vi "API Test.vi"   [LabVIEW 2020]
uses:
  <userlib>/_MGI/User Interface/Progress Bar/Progress Bar.lvclass
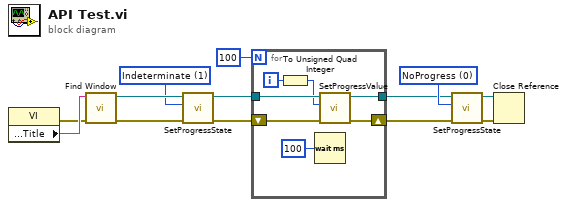
[diagram p0: block diagram]
diagram:
  w12 = 0 items=["NoProgress"=0, "Indeterminate"=1, "Normal"=2, "Error"=4, "Paused"=8] ("State (No Progress)")
  w4 = 1 items=["NoProgress"=0, "Indeterminate"=1, "Normal"=2, "Error"=4, "Paused"=8] ("state")
  n1 = property class="VI"() -> (error out=w1:errorcluster, "Front Panel.Title"=w2:string)  [unwired: 2 in, 1 out]
  n2 = call <userlib>:"Find Window.vi"("error in (no error)"=w1, "Window Title (Callers Window)"=w2) -> ("error out"=w3:errorcluster, "Window Handle"=w5:refnum<k24>)  [unwired: 8 in]
  n3 = call <userlib>:"SetProgressState.vi"("error in (no error)"=w3, "State (No Progress)"=w4, "Window Handle"=w5) -> ("error out"=w6:errorcluster, "dup Window Handle"=w7:refnum<k24>)  [unwired: 7 in]
  n4 = for {
    N: 100 -> [_]
    tunnel: w7 -> [w19]
    shift-right: [w16] -> w10
    shift-left: w6 -> [w20]
    tunnel: [w14] -> w9
    i -> [w18]
    n5 = To Unsigned Quad Integer(1:w18) -> (0:w17:u64)
    n6 = Wait (ms)(milliseconds to wait=u32 100) -> ()  [unwired: 1 out]
    n7 = call <userlib>:"SetProgressValue.vi"("error in (no error)"=w20, "current (0)"=w17, "Window Handle"=w19) -> ("error out"=w16:errorcluster, "dup Window Handle"=w14:refnum<k24>)  [unwired: 7 in]
  }
  n8 = call <userlib>:"SetProgressState.vi"("error in (no error)"=w10, "State (No Progress)"=w12, "Window Handle"=w9) -> ("error out"=w11:errorcluster, "dup Window Handle"=w13:refnum<k24>)  [unwired: 7 in]
  n9 = Close Reference(reference=w13, error in (no error)=w11) -> ()  [unwired: 1 out]
